vi "EventLog.SourceBuffer.Clear.vi"(7 "group":T1=enum."Gui", 8 "error in (no error)":errorcluster) -> (0 "error out":errorcluster)   [LabVIEW 2013]
uses:
  EventLog.SourceBuffer.Action.ctl
  EventLog.EventSource.ctl
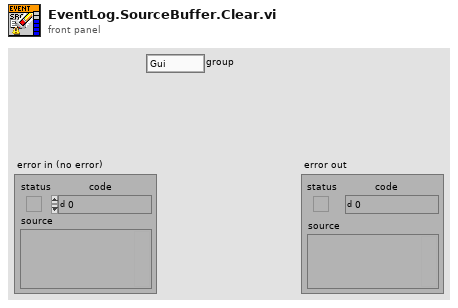
[diagram p1: front panel]
types:
  T1 = typedef "EventLog.EventSource.ctl" = enum16{"All", "Gui", "DB", "Seq", "File", "DIO", "AI", "AO", "IFM", "CPX"}
  T2 = typedef "EventLog.SourceBuffer.Action.ctl" = enum16{"init", "new", "confirm", "check", "get", "get alarms"}
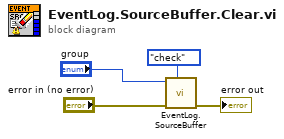
[diagram p0: block diagram]
diagram:
  n1 = call "EventLog.SourceBuffer.vi"("Action"=EventLog.SourceBuffer.Action."check", "error in (no error)"="error in (no error)", 11:"group") -> ("error out"=→"error out":errorcluster)  [unwired: 6 in, 2 out]
